vi "state_machine1.vi"() -> ()   [LabVIEW 2017]
uses:
  typedef_enum_states.ctl
panel:
  in  "?":bool
  in  "?":bool
  out "state":string
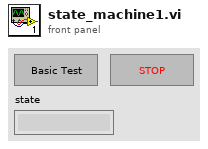
[diagram p1: front panel]
types:
  T1 = typedef "typedef_enum_states.ctl" = enum16{"Init", "Idle", "Basic Test", "Advanced Test", "Notify"}
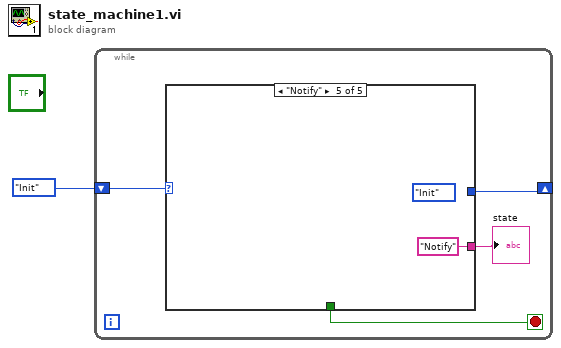
[diagram p0: block diagram]
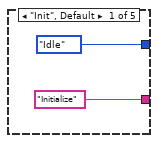
[diagram p2: hidden frame]
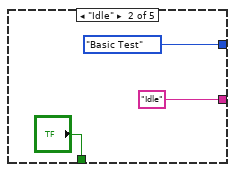
[diagram p3: hidden frame]
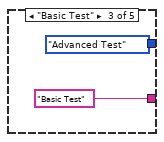
[diagram p4: hidden frame]
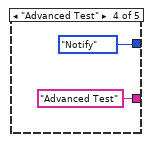
[diagram p5: hidden frame]
diagram:
  n1 = while {
    shift-right: [w2] -> _
    shift-left: typedef_enum_states."Init" -> [w5]
    stop <- w3 stop-if-true
    n2 = case shown="\"Notify\"" w5 {
      tunnel: ["Initialize" "Idle" "Basic Test" "Advanced Test" "Notify"] -> w4
      tunnel: [_ "?" _ _ _] -> w3
      tunnel: [typedef_enum_states."Idle" typedef_enum_states."Basic Test" typedef_enum_states."Advanced Test" typedef_enum_states."Notify" _] -> w2
      frame "Init", Default {
      }
      frame "Idle" {
      }
      frame "Basic Test" {
      }
      frame "Advanced Test" {
      }
      frame "Notify" {
        (unwired) typedef_enum_states."Init"
      }
    }
    "state" <- w4
  }
